vi "FINAL.vi"() -> ()   [LabVIEW 2018]
uses:
  <vilib>/Tufts CEEO ROS for LabVIEW Software/ROS/Code/SubVIs/_ROSControl.ctl
  <vilib>/Tufts CEEO ROS for LabVIEW Software/ROS/Code/SubVIs/_ROSDirection.ctl
  <vilib>/Tufts CEEO ROS for LabVIEW Software/ROS/Code/Console/Servers/ServerSubs/TopicDef.ctl
  <vilib>/Tufts CEEO ROS for LabVIEW Software/ROS/MessageBuilding/std_msgs/subs/stringScalar.vi
panel:
  in  "START/STOP":bool
  out "Robot state":bool
  in  "Manual/\nAUTONOMOUS":bool
  in  "LEFT":bool
  in  "DOWN":bool
  in  "RIGHT":bool
  in  "TOP":bool
  in  "Y POSITION":dbl
  in  "THETA POSITION":dbl
  in  "X POSITION":dbl
  out "ROBOT SPEED":dbl(knob) scale=0.0..10.0
  out "ROS out":T1={"topic port"=0, "Node"="", "topic"="", "type"="", "node port"=0, "error "={"status"=FALSE, "code"=0, "source"=""}, "Direction"=enum."Node", "Update (ms)"=1, "FIFO size"=1}
  out "error out":errorcluster
  out "position graph":cluster{"X":dbl, "Y":dbl}[](graph)
  out "obstacles graph":cluster{"X":dbl, "Y":dbl}[](graph)
  # "Robot state"
  # "MANUAL MODE"
  # "CONTROL\nMODE"
  # "AUTONOMOUS MODE"
  # "MANUAL MODE"
  # "AUTONOMOUS MODE"
  # "ROBOT SPEED"
  # "ROBOT POSITION IN THE MAP"
  # "LASER SCAN PLOT"
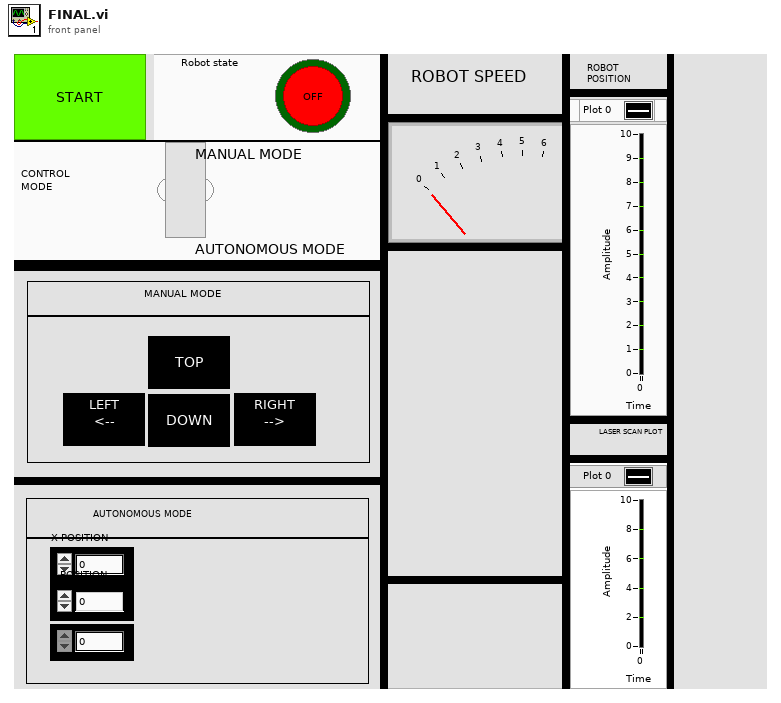
[diagram p1: front panel]
types:
  T1 = typedef "_ROSControl.ctl" = cluster{"topic port":u16, "Node":string, "topic":string, "type":string, "node port":u16, "error ":errorcluster, "Direction":T2, "Update (ms)":u16, "FIFO size":u16}
  T2 = typedef "_ROSDirection.ctl" = enum16{"Node", "Publisher", "Subscriber", "ServiceClient", "ServiceProvider"}
  T3 = typedef "TopicDef.ctl" = cluster{"Topic":string, "Type":string, "Action":T2, "Update (ms)":u16, "queue size":u16}
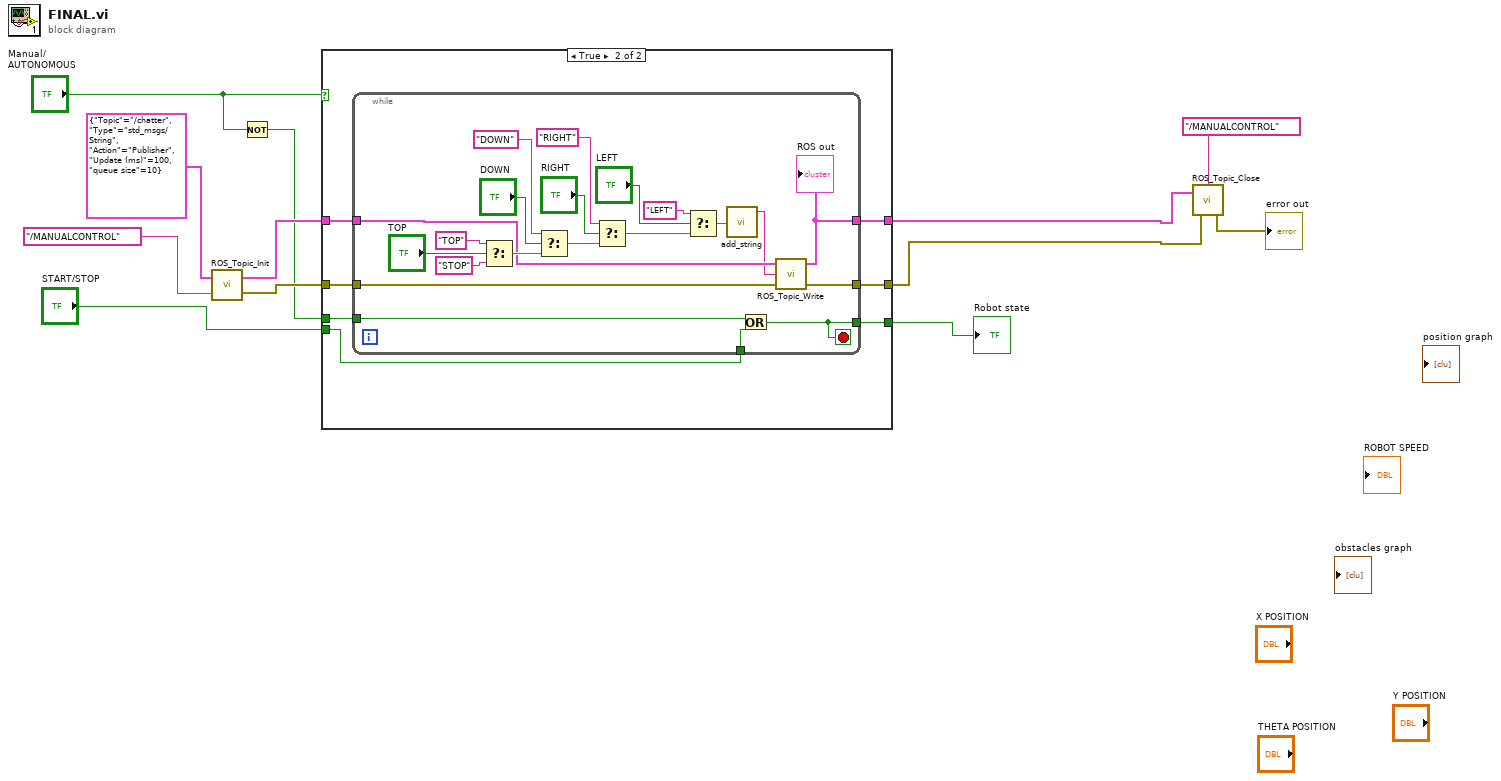
[diagram p0: block diagram]
diagram:
  n1 = call <vilib>:"ROS_Topic_Init.vi"("Definitions"=T3 {"Topic"="/chatter", "Type"="std_msgs/String", "Action"=enum."Publisher", "Update (ms)"=100, "queue size"=10}, "node"="/MANUALCONTROL") -> ("ROS out"=w5:T1, "error out"=w12:errorcluster)  [unwired: 1 in]
  n2 = Not(x="Manual/\nAUTONOMOUS") -> (.not. x?=w3:bool)
  n3 = case shown="True" "Manual/\nAUTONOMOUS" {
    tunnel: w12 -> [w13 w18]
    tunnel: w5 -> [w14 w19]
    tunnel: [w14 w20] -> w7
    tunnel: [w13 w21] -> w6
    tunnel: w3 -> [_ w17]
    tunnel: "START/STOP" -> [_ w16]
    tunnel: [_ w15] -> w1
    frame False {
    }
    frame True {
      n4 = while {
        tunnel: w19 -> [w33]
        tunnel: [w41] -> w20
        tunnel: w18 -> [w32]
        tunnel: [w42] -> w21
        tunnel: w17 -> [w24]
        tunnel: w16 -> [w23]
        tunnel: [w22] -> w15
        stop <- w22 stop-if-true
        n5 = Select(t="TOP", s="TOP", f="STOP") -> (s? t:f=w40:string)
        n6 = Select(t="DOWN", s="DOWN", f=w40) -> (s? t:f=w39:string)
        n7 = Select(t="RIGHT", s="RIGHT", f=w39) -> (s? t:f=w29:string)
        n8 = Select(t="LEFT", s="LEFT", f=w29) -> (s? t:f=w26:string)
        n9 = call-poly <vilib>:"add_string.vi"("String"=w26) -> ("msg out"=w25:string)  [unwired: 4 in]
        n10 = Or(x=w24, y=w23) -> (x .or. y?=w22:bool)
        n11 = call <vilib>:"ROS_Topic_Write.vi"("error in (no error)"=w32, "Msg in"=w25, "ROS in"=w33) -> ("error out"=w42:errorcluster, "ROS out"=w41:T1)  [unwired: 1 in]
        "ROS out" <- w41
      }
    }
  }
  "Robot state" <- w1
  n12 = call <vilib>:"ROS_Topic_Close.vi"("error in"=w6, "ROS in"=w7, "node"="/MANUALCONTROL") -> ("error out"=→"error out":errorcluster)  [unwired: 1 in]
